vi "FT10_Fornax Mono2 Cut Activate Port Command.vi"(10 "Mono2 Cut Activate":T1, 11 "TCP Network Connection in":refnum<k5>) -> (3 "TCP Network Connection out":refnum<k5>)   [LabVIEW 2015]
uses:
  Controls/Control_Fornax Mono2 Cut Activate Port Bool.ctl
  Controls/Control_Fornax Generator.ctl
  Controls/Control_Fornax Source ID.ctl
  Controls/Control_Fornax Switch ID.ctl
  Controls/Control_Fornax Energy Channel ID.ctl
  Controls/Control_Fornax Switch State.ctl
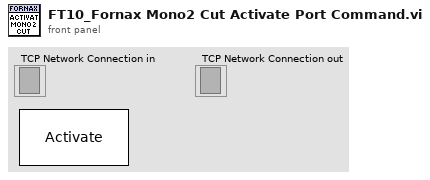
[diagram p1: front panel]
types:
  T1 = typedef "Control_Fornax Mono2 Cut Activate Port Bool.ctl" = bool
  T2 = typedef "Control_Fornax Switch State.ctl" = enum16{"SWITCH_STATE_NULL  ", "SWITCH_STATE_PRESSED  ", "SWITCH_STATE_RELEASED  ", "NUM_SWITCH_STATES  "}
  T3 = typedef "Control_Fornax Energy Channel ID.ctl" = enum16{"EC_MONO_1  ", "EC_BIPOLAR  ", "EC_MONO_2  ", "EC_ADVANCED  ", "EC_ADVANCED_ECUT  ", "EC_ADVANCED_DCUT  ", "EC_SHARED_COAG  ", "EC_INTERNAL_BIP_CAL  "}
  T4 = typedef "Control_Fornax Switch ID.ctl" = enum16{"SWITCH_ID_NONE  ", "SWITCH_ID_CUT  ", "SWITCH_ID_VMODE  ", "SWITCH_ID_COAG  ", "SWITCH_ID_LIGASURE  ", "SWITCH_ID_BIPOLAR  ", "SWITCH_ID_STAPLER_CLOSE  ", "SWITCH_ID_STAPLER_OPEN  ", "SWITCH_ID_CARDIOBLATE_BIPOLAR  ", "SWITCH_ID_CARDIOBLATE_BIPOLAR_TOUCHSCREEN  ", "SWITCH_ID_CARDIOBLATE_MONOPOLAR  ", "SWITCH_ID_CARDIOBLATE_MONOPOLAR_TOUCHSCREEN  ", "SWITCH_ID_ULTRASONIC_BTN1  ", "SWITCH_ID_ULTRASONIC_BTN2  ", "SWITCH_ID_MAX  "}
  T5 = typedef "Control_Fornax Source ID.ctl" = enum16{"SWITCH_SOURCE_UNKNOWN  ", "SWITCH_SOURCE_HANDSWITCH  ", "SWITCH_SOURCE_FOOTSWITCH  ", "SWITCH_SOURCE_AUTO_BIPOLAR  ", "SWITCH_SOURCE_CARDIOBLATE  ", "SWITCH_SOURCE_SCREEN  ", "NUM_SWITCH_SOURCES  "}
  T6 = typedef "Control_Fornax Generator.ctl" = string
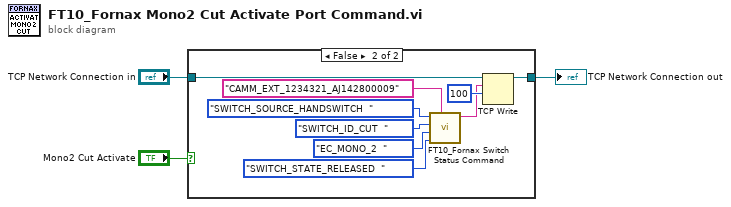
[diagram p0: block diagram]
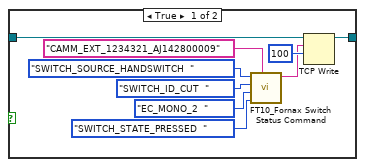
[diagram p2: hidden frame]
diagram:
  n1 = case shown="False" "Mono2 Cut Activate" {
    tunnel: "TCP Network Connection in" -> [w12 w21]
    tunnel: [w11 w20] -> w3
    frame True {
      n2 = call "FT10_Fornax Switch Status Command.vi"("Generator"=T6 "CAMM_EXT_1234321_AJ142800009", "Switch State"=Control_Fornax_Switch_State."SWITCH_STATE_PRESSED  ", "Energy Channel ID"=Control_Fornax_Energy_Channel_ID."EC_MONO_2  ", "Switch ID"=Control_Fornax_Switch_ID."SWITCH_ID_CUT  ", "Source ID"=Control_Fornax_Source_ID."SWITCH_SOURCE_HANDSWITCH  ") -> ("JSON Command"=w4:string)  [unwired: 6 in]
      n3 = TCP Write(connection ID=w12, data in=w4, 9:100 ("timeout ms (25000)")) -> (connection ID out=w11:refnum<k5>)  [unwired: 1 in, 2 out]
    }
    frame False {
      n4 = call "FT10_Fornax Switch Status Command.vi"("Generator"=T6 "CAMM_EXT_1234321_AJ142800009", "Switch State"=Control_Fornax_Switch_State."SWITCH_STATE_RELEASED  ", "Energy Channel ID"=Control_Fornax_Energy_Channel_ID."EC_MONO_2  ", "Switch ID"=Control_Fornax_Switch_ID."SWITCH_ID_CUT  ", "Source ID"=Control_Fornax_Source_ID."SWITCH_SOURCE_HANDSWITCH  ") -> ("JSON Command"=w13:string)  [unwired: 6 in]
      n5 = TCP Write(connection ID=w21, data in=w13, 9:100 ("timeout ms (25000)")) -> (connection ID out=w20:refnum<k5>)  [unwired: 1 in, 2 out]
    }
  }
  "TCP Network Connection out" <- w3
